vi "IETS_Tool_14_0805_bias_correct_neg_setpoints.vi"() -> ()   [LabVIEW 2013]
doc: "I. Description:\nThis example demonstrates how to continuously acquire and generate data at the same time, synchronized with one another.\n\nII. Instructions for Running:\n1. Select the physical channel to correspond to where your signal is input on the DAQ device. Also, select the corresponding channel for where your signal is being generated.\n2. Enter the minimum and maximum voltage ranges.\nNote: For better accuracy try to match the input range to the expected voltage level of the measured signal.\n3. Set the sample rate of the acquisition.\nNote: The rate should be at least twice as fast as the maximum frequency component of the signal being acquired. \n6. Select the Rate for the generation\n7. Select what type of signal to generate and the amplitude.\nNote: This example requires two DMA channels to run. If your hardware does not support two DMA channels, you need to set the Data Transfer Mechanism property for the Analog Output Task to use \"Interrupts\". The Data Transfer Mechanism property is located in the DAQmx Channel Property hierarchy at:\n\nDAQmx Channel Property Node>>Analog Output>>General Properties>>Advanced>>Data Transfer and Memory>>Data Transfer Mechanism\n\nRefer to your device documentation to determine how many DMA channels are supported for your hardware.\n\nIII. Block Diagram Steps:\n1. Create an analog input voltage channel. Also, create an analog output voltage channel.\n2. Set the rate for the sample clock. Additionally, define the sample mode to be continuous. Also, set the sample clock rate for the signal generation.\n2a. Call the Get Terminal Name with Device Prefix VI. This will take a Task and a terminal and create a properly formatted device + terminal name to use as the source of the Trigger.\n3. Define the parameters for a Digital Edge Start Trigger. Set the Analog output to trigger off the AI Start Trigger. This is an internal trigger signal.\n4. Use the Basic Function Generator VI to create the signal to be generated.\n5. Call the Start VI to arm the two functions. Make sure the analog output is armed before the analog input. This will ensure both will start at the same time.\n6. Read the waveform data in a loop until the user hits the stop button or an error occurs. The Is Task Done? VI is used to check for errors in the Analog Output Task.\n7. Call the Clear VI to Clear the Task\n8. Use the popup dialog box to display an error if any.\n\nIV. I/O Connections Overview:\nMake sure your signal input/output terminals match the Physical Channel I/O controls."
uses:
  <vilib>/Utility/error.llb/DialogType.ctl
  <vilib>/DAQmx/write.llb/DAQmx Write (Analog 2D DBL NChan NSamp).vi
  <vilib>/DAQmx/read.llb/DAQmx Read (Analog 1D DBL NChan 1Samp).vi
  <vilib>/DAQmx/write.llb/DAQmx Write (Analog DBL 1Chan 1Samp).vi
  <vilib>/DAQmx/read.llb/DAQmx Read (Analog DBL 1Chan 1Samp).vi
  <vilib>/Analysis/baseanly.llb/Mean (DBL).vi
  <vilib>/DAQmx/write.llb/DAQmx Write (Analog 1D DBL NChan 1Samp).vi
  <vilib>/DAQmx/create/channels.llb/DAQmx Create Channel (AO-Voltage-Basic).vi
  <vilib>/DAQmx/create/channels.llb/DAQmx Create Channel (AI-Voltage-Basic).vi
  <vilib>/DAQmx/configure/timing.llb/DAQmx Timing (Sample Clock).vi
  <vilib>/DAQmx/configure/trigger.llb/DAQmx Start Trigger (Digital Edge).vi
  <vilib>/DAQmx/miscellaneous.llb/DAQmx Fill In Error Info.vi
  <vilib>/Utility/file.llb/Write To Spreadsheet File (DBL).vi
  pid/pid.llb/PID (DBL).vi
  pid/pid.llb/PID Output Rate Limiter (DBL).vi
  <vilib>/ptbypt/NI_PtbyPt.lvlib
  <resource>/objmgr/daqmx.rc
  <vilib>/Analysis/NI_AALBase.lvlib
panel:
  in  "Bias Offset Correct":dbl
  out "Bias Sweep":dbl[](graph)
  out "element":dbl
  out "mean":dbl format="%.6f"
  out "size(s)":i32
  out "Numeric":i32
  in  "PID":bool=TRUE caption="Step Z"
  in  "Tab Control":enum32{"PID Controller", "Tapping Controls"}(tab)=enum."Tapping Controls"
  in  "Proportional Gain":dbl=0.0001
  in  "Integral Gain":dbl=1e-07
  in  "Differential Gain":dbl=1e-05
  in  "Setpoint":dbl=0.1
  in  "Piezo Delta rate":dbl=1000.0
  in  "Min Current":dbl=0.002
  in  "Max Current":dbl=10.2
  in  "Ramp Rate":dbl=20.0
  in  "Make Contact":i32=1200
  in  "Break Contact":i32=500
  in  "Step Length":i32=100
  in  "Step Max":dbl=0.3
  in  "Step Min":dbl=0.05
  out "Tapping Stop":bool
  out "Case":i32
  in  "Contact Cycles":i32
  in  "Tapping":bool caption="Step Z"
  out "x/y":dbl
  out "Waveform Chart":dbl(graph)
  in  "Piezo Control":dbl(slide) min=-10.0 max=10.0 step=0.001 scale=-10.0..10.0
  in  "Manual Z":bool caption="Step Z"
  in  "Sweep Amplitude":dbl=1.0
  in  "Stop Sweep":bool
  out "Connections 2":string="AI0=Current\nAI1=Bias\nAI2=dI/dV\nAI3=d2I/dV2\nAI4=X-Axis\nAI5=Z-Axis\n"
  out "Connections":string="AO0=Bias\nAO1=Z-axis\nAO2=X-Axis\nAO3=NA"
  out "Save Indicator":bool
  in  "Z-Direction":bool caption="Step Z"
  in  "Update Bias":bool
  in  "Save IV":bool
  in  "Save Decay":bool
  in  "Sweep Bias":bool
  in  "Step Z":bool
  in  "Comment":string="Molecule=TP4\nGain=10nA\nBias Gain=div/1\nSweep Freq.=0.0008Hz\nRef. Bias=4mV\nRef. Freq=2.977kHz\nGain LIA1=2mV\nTC LIA1=1s\nGain LIA2=5mV\nTC LIA2=1s\nLIA1=EGG\nLIA2=SRS\nEGG is driving(possible 5mV offset)"
  in  "Number Recorded":i32
  in  "DATA Filename":string="Data_"
  in  "Data Directory":path=path "E:/Research/Data"
  out "Current Decay":cluster{dbl[], dbl[]}(graph)
  out "d2I/dV2":cluster{dbl[], dbl[]}(graph)
  out "dI/dV":cluster{dbl[], dbl[]}(graph)
  out "IV":cluster{dbl[], dbl[]}(graph)
  in  "# Samples":i32=2000
  in  "Frequency (Hz)":dbl=1.0
  out "Measurement 2":cluster{i32, dbl, dbl[]}(graph) caption="Measurement"
  out "Actual Update Generation Rate 2":dbl=5000.0 caption="Actual Update Generation Rate" format="%0.2f"
  in  "stop 3":bool
  in  "Bias":dbl=0.1 caption="Bias Start Point" step=0.1 format="%_3g"
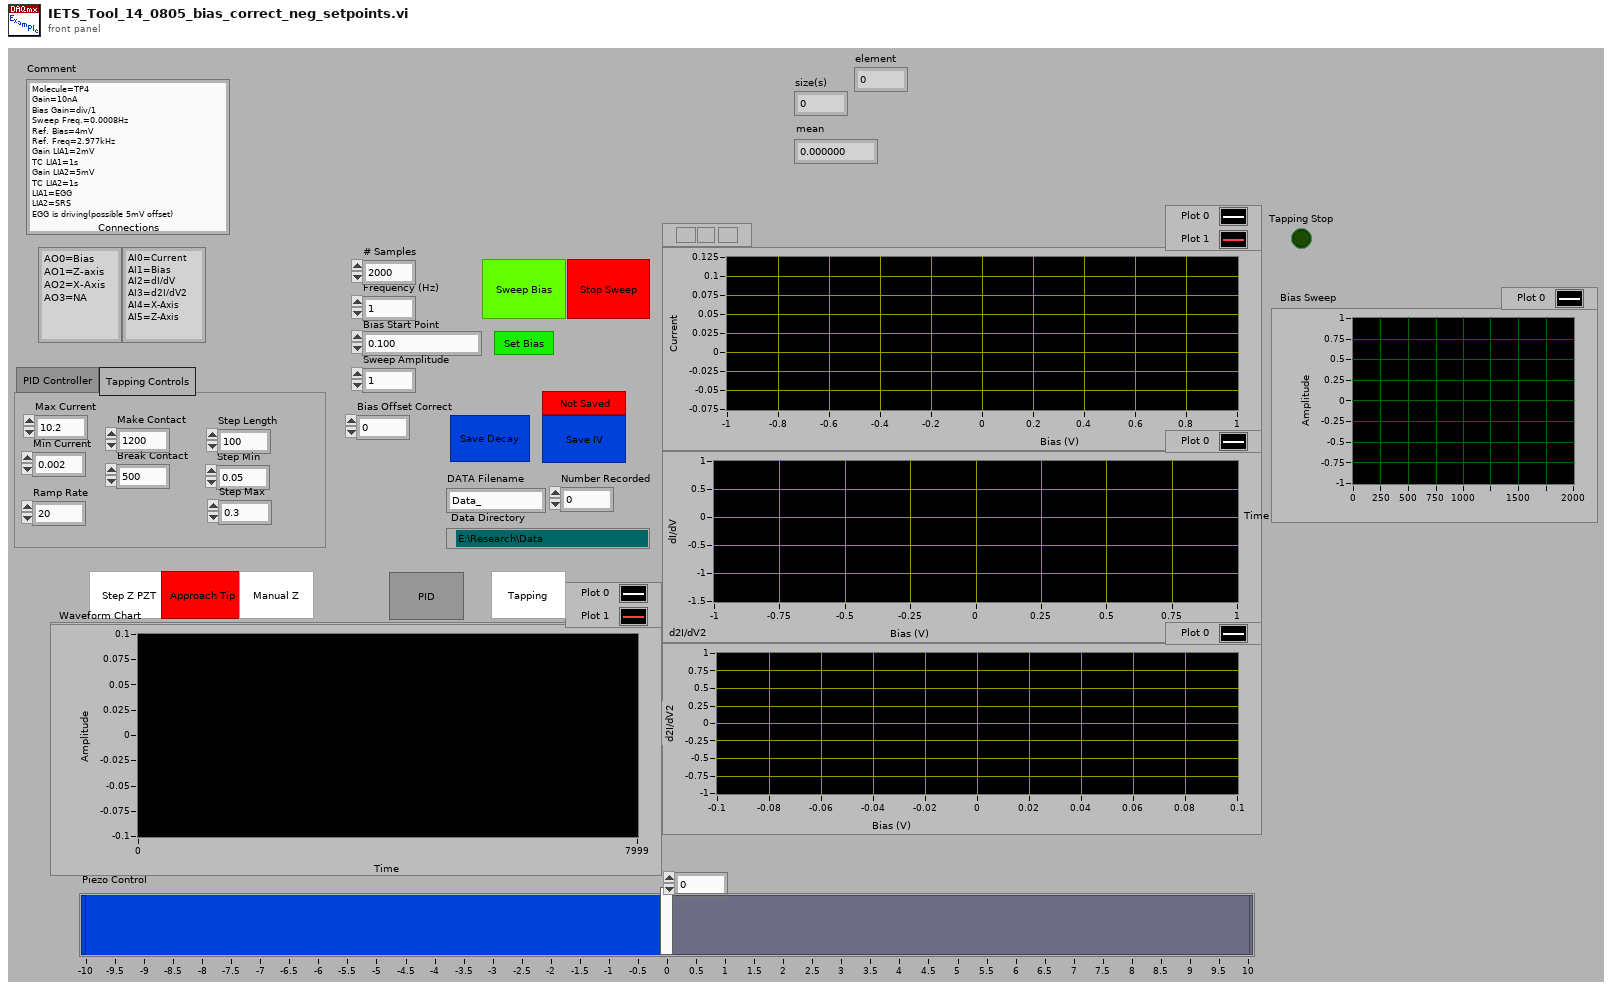
[diagram p1: front panel]
types:
  T1 = enum16{"open", "replace", "create", "open or create", "replace or create", "replace or create with confirmation"}
  T2 = typedef "DialogType.ctl" = u16
  T3 = cluster{"Proportional Gain":dbl, "Integral Gain ":dbl, "Differential Gain":dbl}
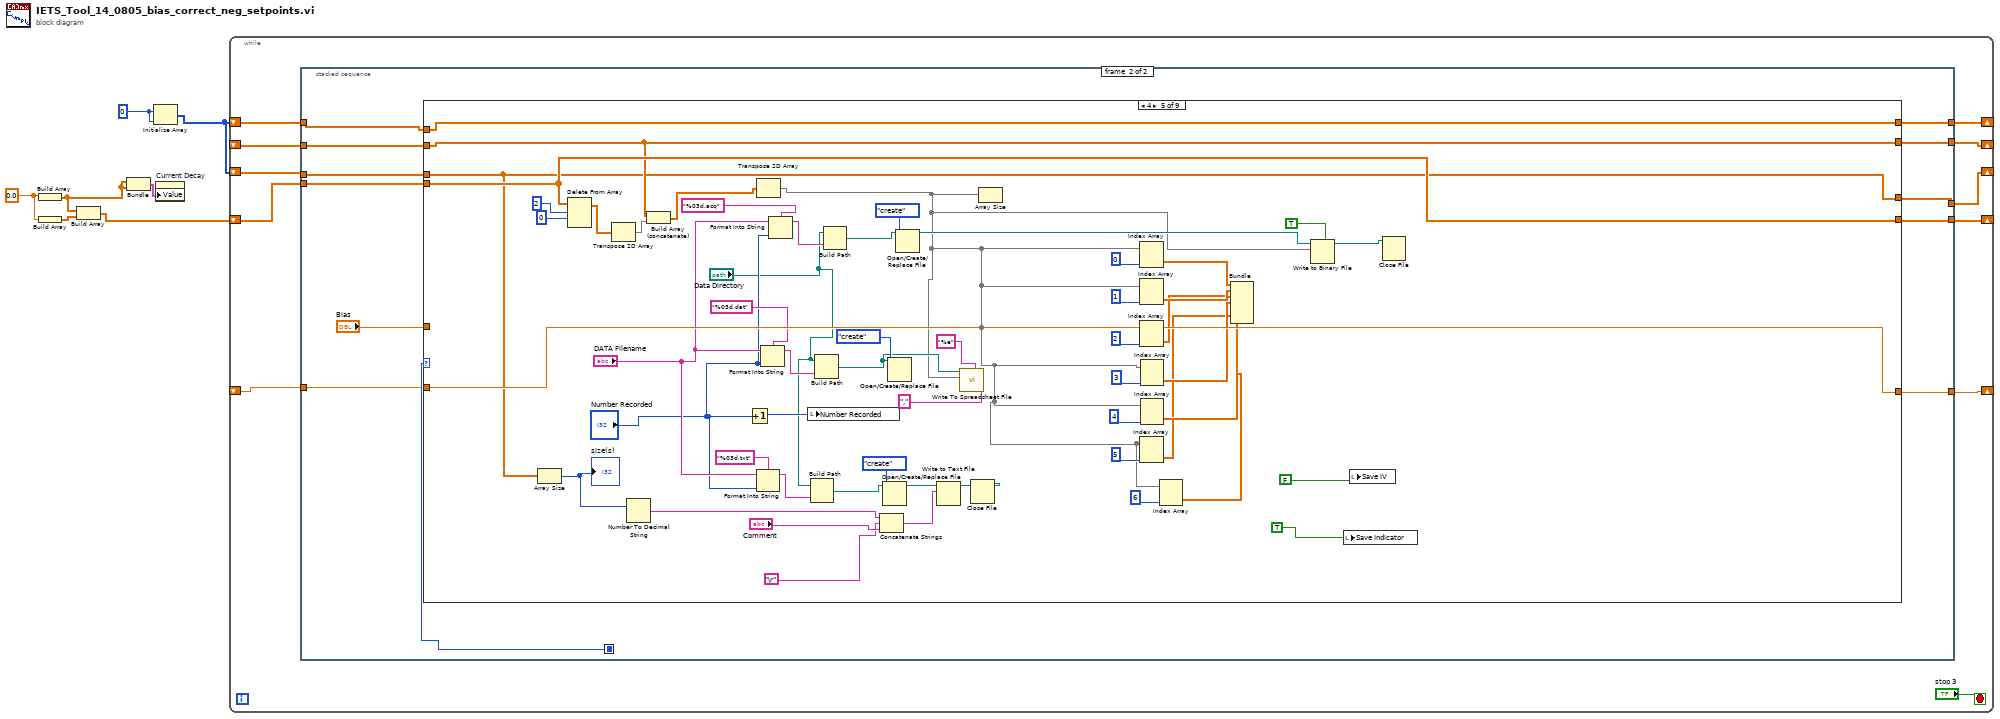
[diagram p0: block diagram]
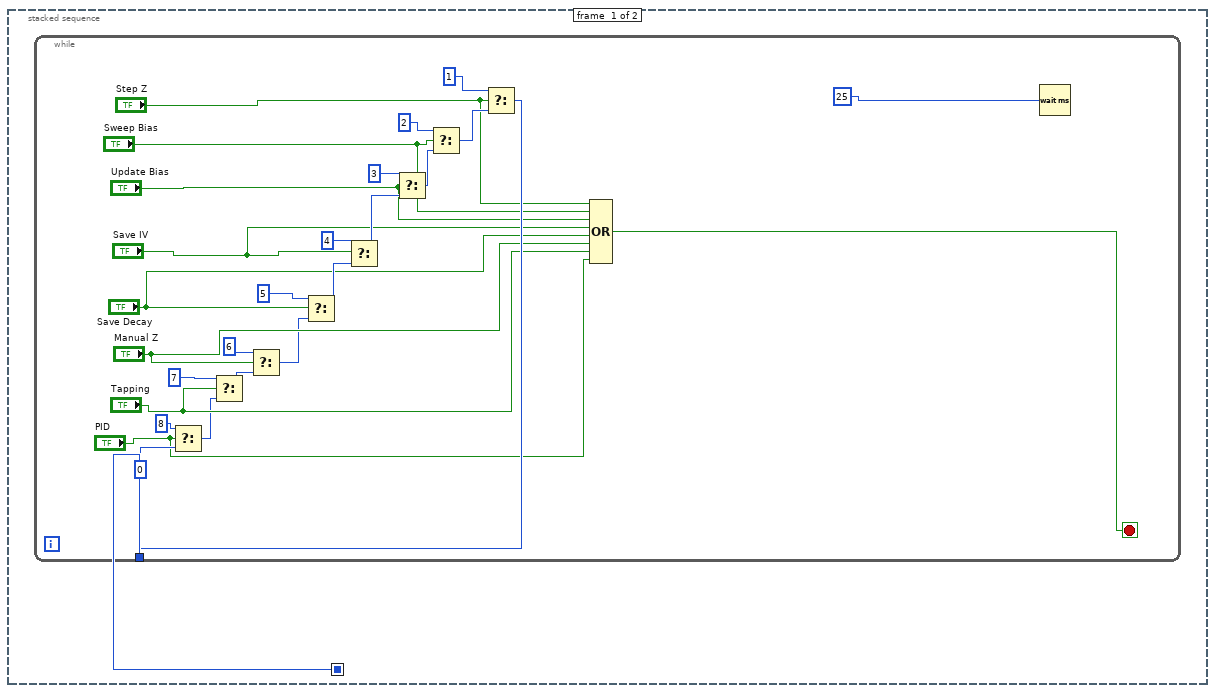
[diagram p2: hidden frame]
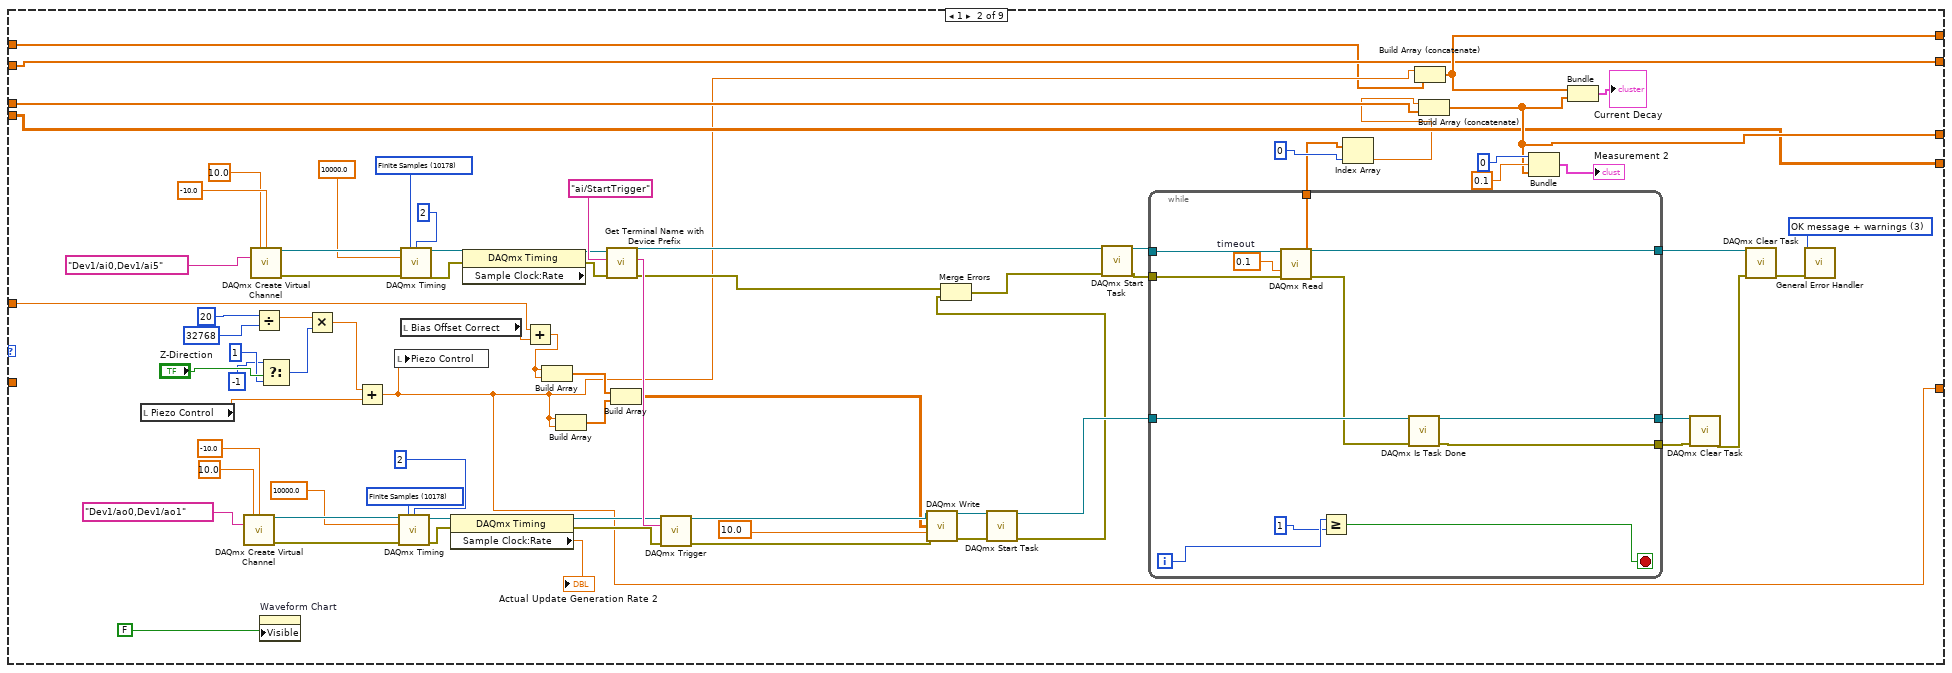
[diagram p4: hidden frame]
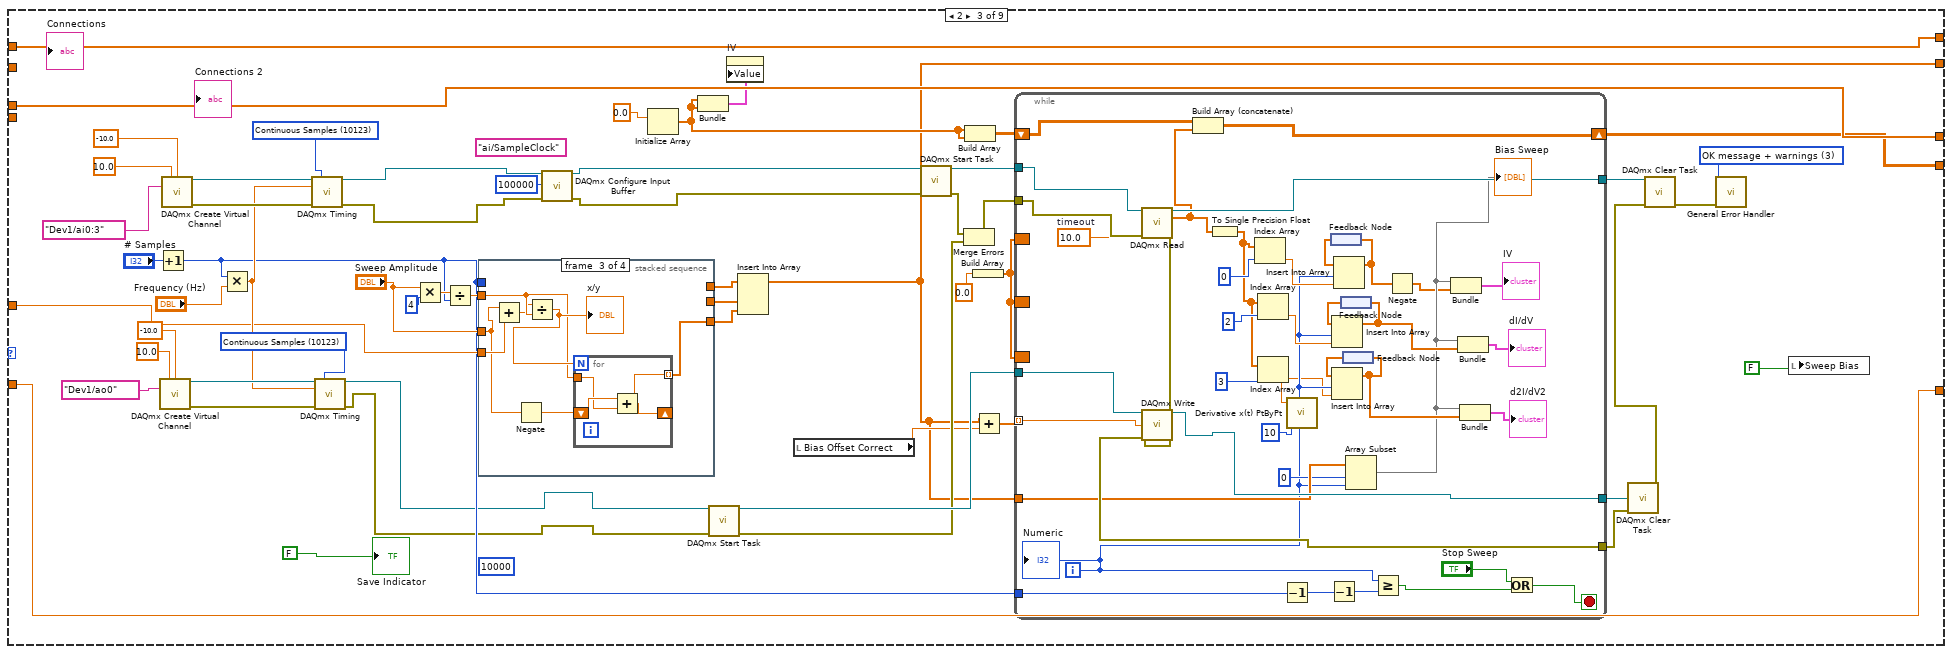
[diagram p5: hidden frame]
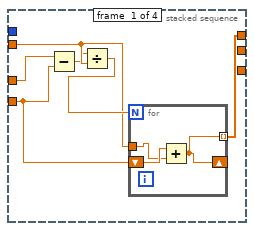
[diagram p6: hidden frame]
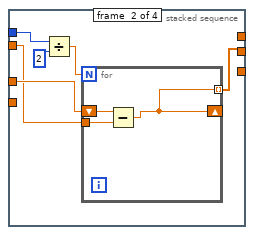
[diagram p7: hidden frame]
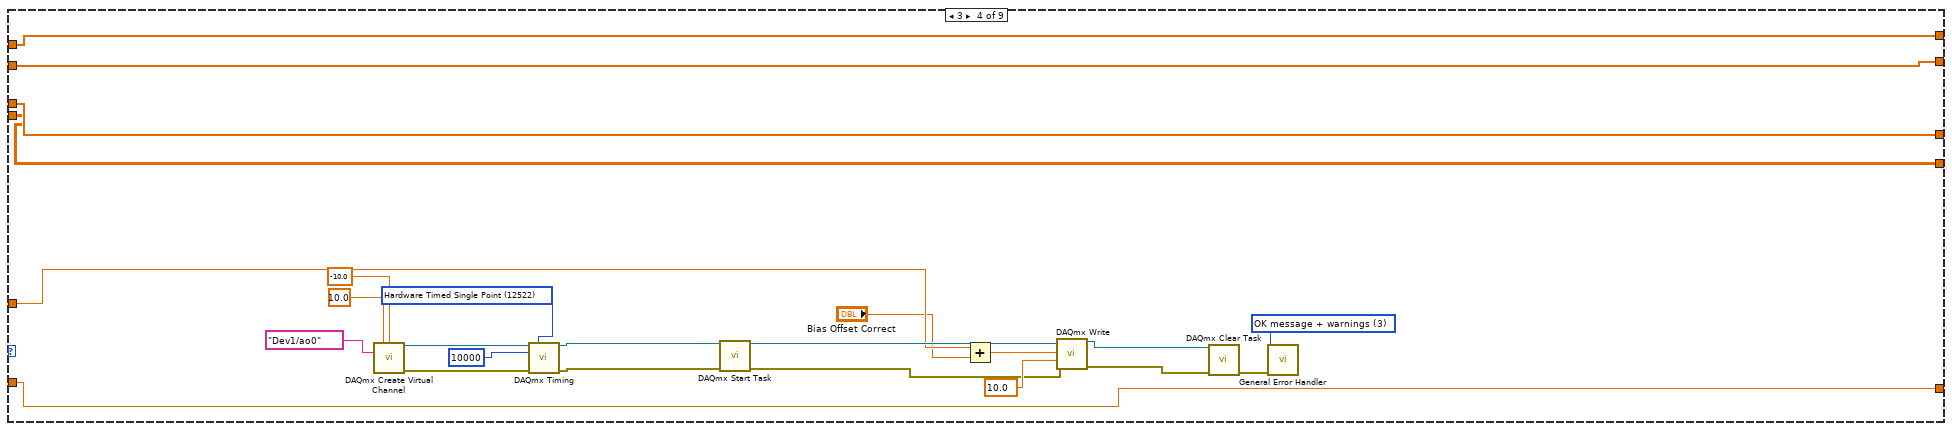
[diagram p9: hidden frame]
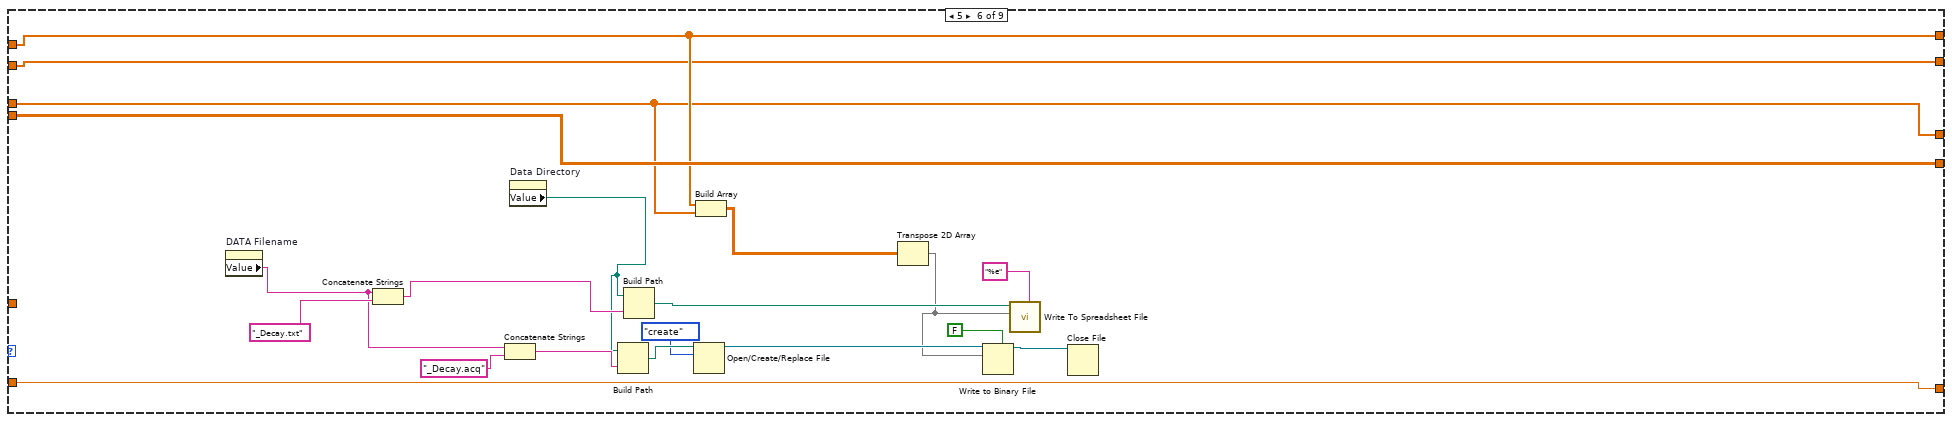
[diagram p10: hidden frame]
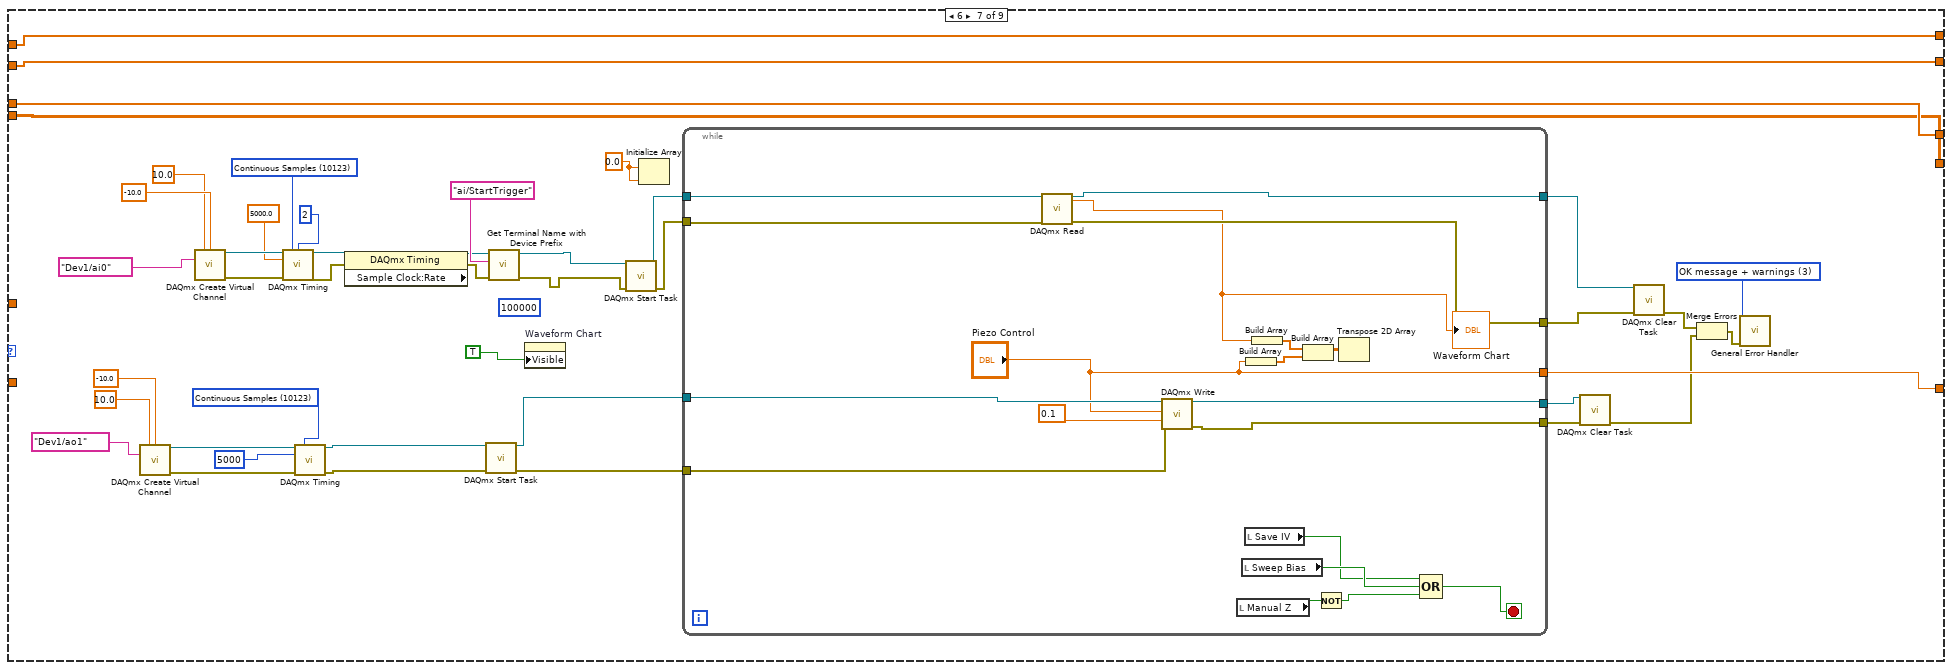
[diagram p11: hidden frame]
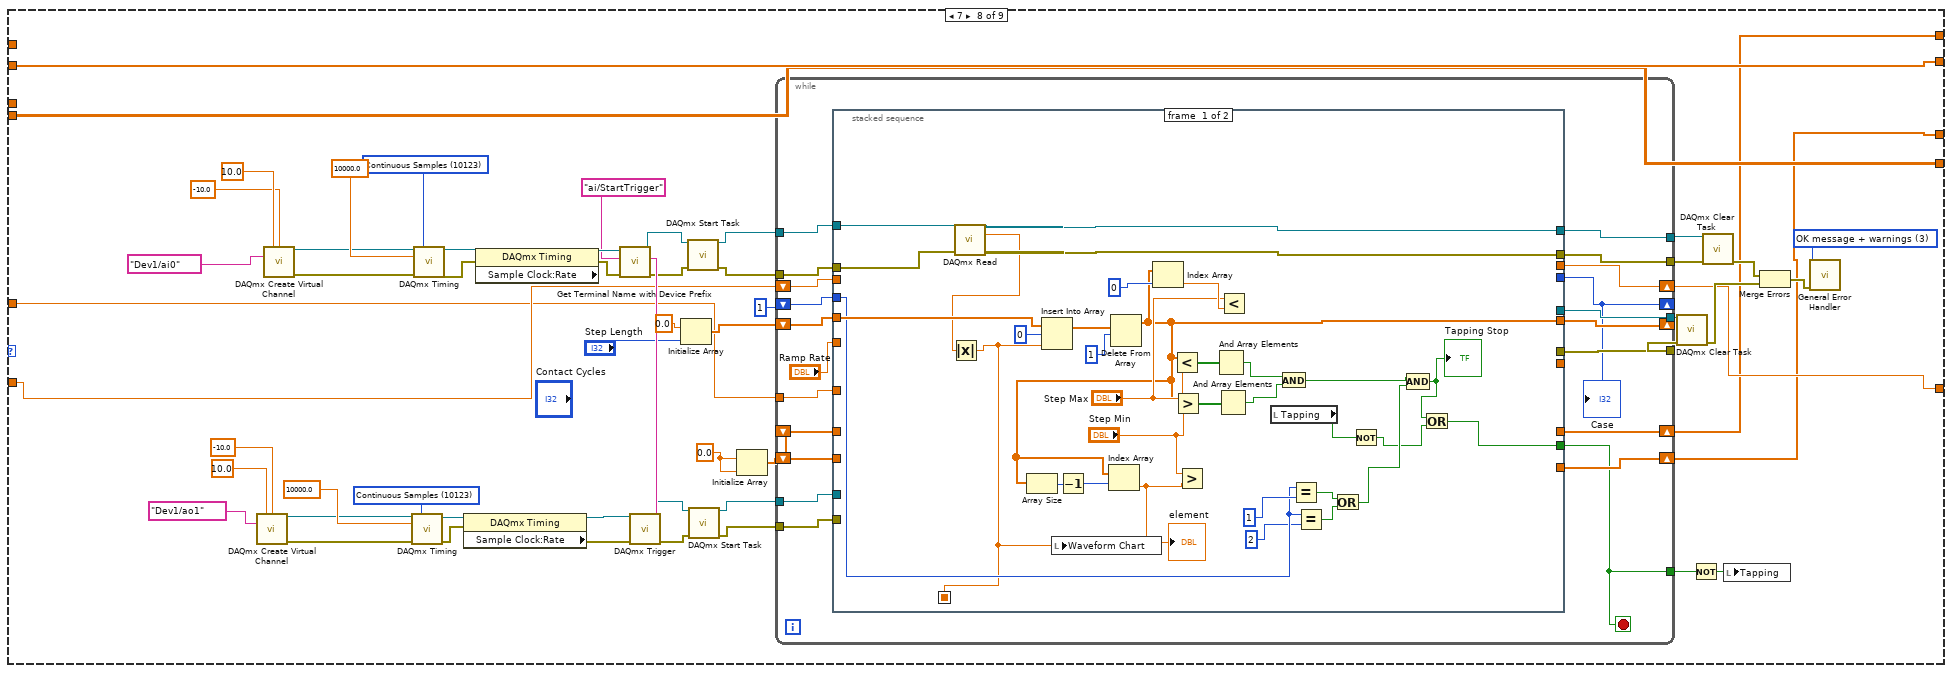
[diagram p12: hidden frame]
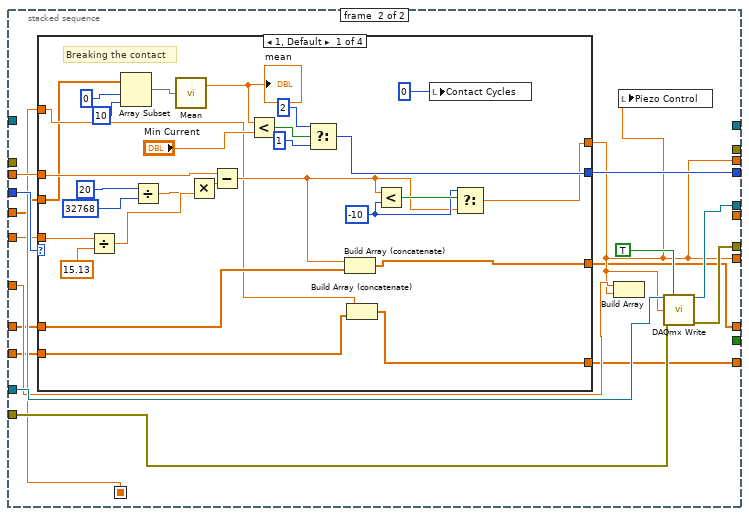
[diagram p13: hidden frame]
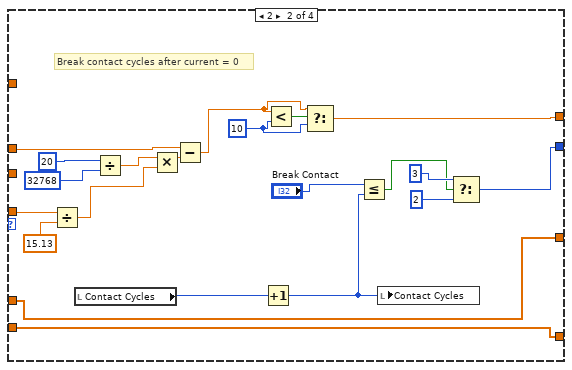
[diagram p14: hidden frame]
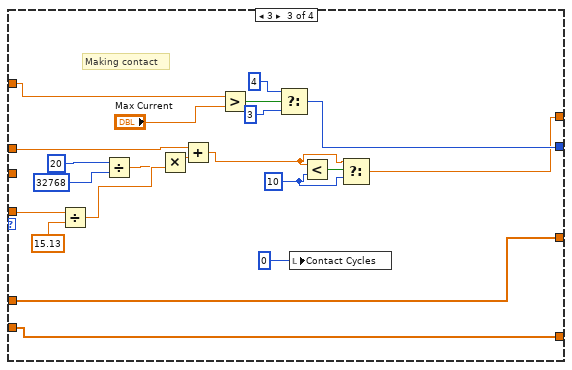
[diagram p15: hidden frame]
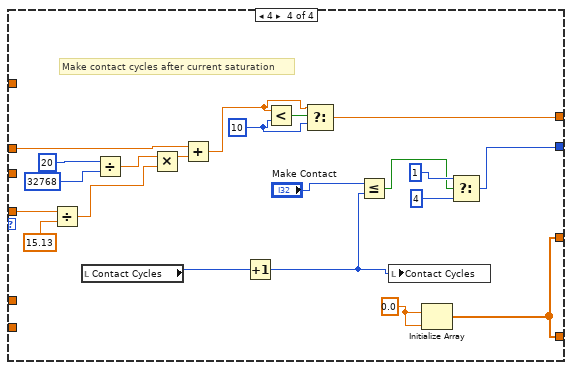
[diagram p16: hidden frame]
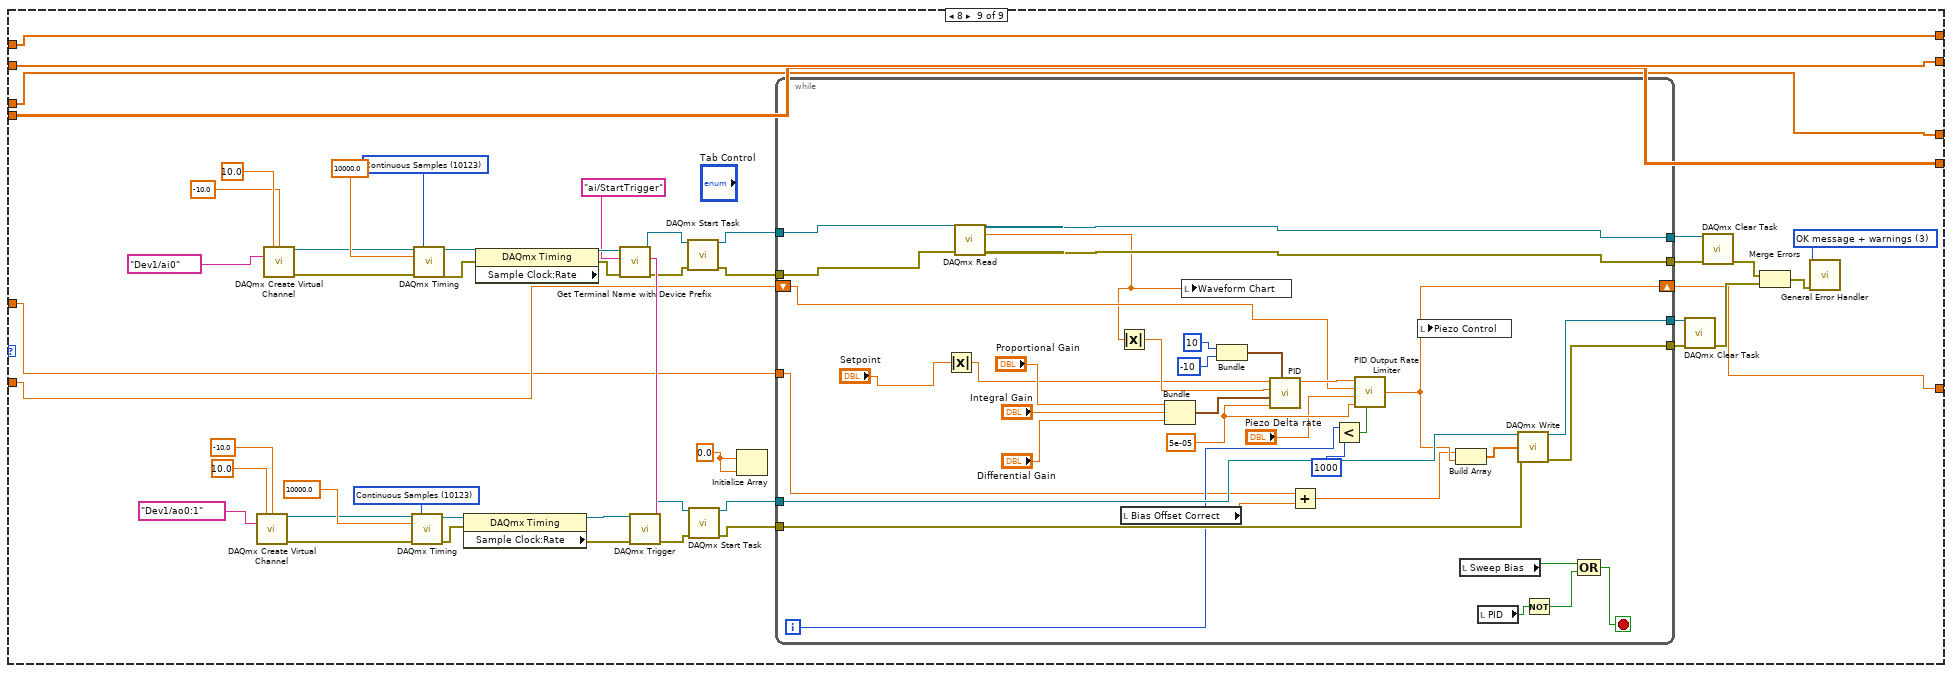
[diagram p17: hidden frame]
diagram:
  w2 = 0
  w7 = 0.0
  n1 = Build Array(w7) -> (w4:dbl[])
  n2 = Build Array(w7) -> (w6:dbl[])
  n3 = Build Array(w4, w6) -> (w5:dbl[][])
  n4 = Bundle(w4, w4) -> (w3:cluster{dbl[], dbl[]})  [unwired: 1 in]
  n5 = Initialize Array(w2, w2) -> (w1:i32[])
  n6 = property on="Current Decay" class="XYGraph (strict)"("Value"=w3) -> ()  [unwired: 2 in, 2 out]
  n7 = while {
    shift-right: [w16] -> _
    shift-left: w1 -> [w17]
    shift-right: [w14] -> _
    shift-left: w1 -> [w15]
    shift-right: [w12] -> _
    shift-left: _ -> [w13]
    shift-right: [w10] -> _
    shift-left: w5 -> [w11]
    shift-right: [w8] -> _
    shift-left: _ -> [w9]
    stop <- "stop 3" stop-if-true
    n8 = stacked-sequence {
      seq-local: [w19 _] -> [_ w58]
      tunnel: w17 -> [_ w57]
      tunnel: [_ w56] -> w16
      tunnel: w15 -> [_ w54]
      tunnel: [_ w53] -> w14
      tunnel: w13 -> [_ w52]
      tunnel: [_ w47] -> w12
      tunnel: w11 -> [_ w51]
      tunnel: [_ w50] -> w10
      tunnel: w9 -> [_ w49]
      tunnel: [_ w48] -> w8
      frame #0 {
        n9 = while {
          tunnel: [w37] -> w19
          stop <- w36 stop-if-true
          n10 = Select(t=8, s="PID", f=0) -> (s? t:f=w23:i32)
          n11 = Select(t=7, s="Tapping", f=w23) -> (s? t:f=w25:i32)
          n12 = Select(t=6, s="Manual Z", f=w25) -> (s? t:f=w26:i32)
          n13 = Select(t=5, s="Save Decay", f=w26) -> (s? t:f=w42:i32)
          n14 = Select(t=4, s="Save IV", f=w42) -> (s? t:f=w41:i32)
          n15 = Select(t=3, s="Update Bias", f=w41) -> (s? t:f=w39:i32)
          n16 = Select(t=2, s="Sweep Bias", f=w39) -> (s? t:f=w46:i32)
          n17 = Select(t=1, s="Step Z", f=w46) -> (s? t:f=w37:i32)
          n18 = Compound Arithmetic op=OR("Step Z", "Sweep Bias", "Update Bias", "Save IV", "Save Decay", "Manual Z", "Tapping", "PID") -> (w36:bool)
          n19 = Wait (ms)(milliseconds to wait=25) -> ()  [unwired: 1 out]
        }
      }
      frame #1 {
        n20 = case shown="4" w58 {
          tunnel: w57 -> [w63 w70 w191 w283 w303 w370 w415 _ w655]
          tunnel: [w63 w83 w191 w283 w303 w370 w415 w441 w655] -> w56
          tunnel: "Bias" -> [_ w66 w176 w277 _ _ _ w447 w654]
          tunnel: w54 -> [w62 w67 w188 w284 w350 w371 w417 _ w656]
          tunnel: [w62 w84 w188 w284 w350 w371 w417 w442 w656] -> w53
          tunnel: w52 -> [w61 _ w187 w282 w349 w372 _ w448 w663]
          tunnel: [w61 w68 w187 w282 w349 w372 w386 w443 w660] -> w47
          tunnel: w51 -> [w60 w81 _ w280 w329 w373 w414 w445 w661]
          tunnel: [w60 w81 w168 w280 w329 w373 w414 w445 w661] -> w50
          tunnel: [w59 w76 w151 w279 w327 w355 w416 w446 w662] -> w48
          tunnel: w49 -> [w59 w76 _ w279 w327 w355 w416 w446 w662]
          frame 0, Default {
          }
          frame 1 {
            w118 = T2 3 items=["no dialog", "OK message", "continue or stop message", "OK message + warnings", "continue/stop + warnings"] ("type of dialog (OK msg:1)")
            w130 = 10178 items=["Finite Samples"=10178, "Continuous Samples"=10123] ("sample mode")
            w135 = 10178 items=["Finite Samples"=10178, "Continuous Samples"=10123] ("sample mode")
            n21 = local read "Piezo Control"() -> (w71:dbl)
            n22 = call-poly <vilib>:"DAQmx Create Virtual Channel.vi"("maximum value"=10.0 ("maximum value 2"), "minimum value"=-10.0 ("minimum value 2"), "physical channels"=tag "Dev1/ao0,Dev1/ao1" ("physical channels 2")) -> ("task out"=w129:refnum<k21>, "error out"=w128:errorcluster)  [unwired: 11 in]
            n23 = call-poly <vilib>:"DAQmx Create Virtual Channel.vi"("maximum value"=10.0 ("Maximum Value 2"), "minimum value"=-10.0 ("Minimum Value 2"), "physical channels"=tag "Dev1/ai0,Dev1/ai5" ("Physical Channel 2")) -> ("task out"=w133:refnum<k21>, "error out"=w134:errorcluster)  [unwired: 11 in]
            n24 = Divide(x=20, y=32768) -> (x/y=w80:dbl)
            n25 = property on="Waveform Chart" class="WFChart (strict)"("Visible"=FALSE) -> ()  [unwired: 2 in, 2 out]
            n26 = Select(t=-1 ("f"), s="Z-Direction", f=1) -> (s? t:f=w78:i32)
            n27 = Multiply(x=w80, y=w78) -> (x*y=w79:dbl)
            n28 = Add(x=w79, y=w71) -> (x+y=w68:dbl)
            n29 = local write "Piezo Control"(w68) -> ()
            n30 = call-poly <vilib>:"DAQmx Timing.vi"("task/channels in"=w129, "sample mode"=w130, "samples per channel"=2, "rate"=10000.0 ("rate 2"), "error in"=w128) -> ("task out"=w113:refnum<k21>, "error out"=w112:errorcluster)  [unwired: 9 in]
            n31 = call-poly <vilib>:"DAQmx Timing.vi"("task/channels in"=w133, "sample mode"=w135, "samples per channel"=2, "rate"=10000.0 ("Rate 2"), "error in"=w134) -> ("task out"=w107:refnum<k21>, "error out"=w106:errorcluster)  [unwired: 9 in]
            n32 = local read "Bias Offset Correct"() -> (w65:dbl)
            n33 = property class="DAQmx Timing"(reference=w113, error in=w112) -> (reference out=w114:refnum<k21>, error out=w111:errorcluster, "Sample Clock:Rate"=→"Actual Update Generation Rate 2":dbl)
            n34 = property class="DAQmx Timing" props=["Sample Clock:Rate"](reference=w107, error in=w106) -> (reference out=w105:refnum<k21>, error out=w104:errorcluster)  [unwired: 1 out]
            n35 = Add(x=w66, y=w65) -> (x+y=w64:dbl)
            n36 = Build Array(w64, w64) -> (w91:dbl[])
            n37 = Build Array(w68, w68) -> (w90:dbl[])
            n38 = call "Get Terminal Name with Device Prefix.vi"("error in (no error)"=w104, "Local Terminal Name"="ai/StartTrigger" ("terminal"), "task/channels in"=w105) -> ("error out"=w110:errorcluster, "Terminal Name with Device Prefix"=w115:tag, "task out"=w95:refnum<k21>)  [unwired: 6 in]
            n39 = Build Array(w91, w90) -> (w89:dbl[][])
            n40 = call-poly <vilib>:"DAQmx Trigger.vi"("task/channels in"=w114, "source"=w115, "error in"=w111) -> ("task out"=w120:refnum<k21>, "error out"=w121:errorcluster)  [unwired: 11 in]
            n41 = call-poly <vilib>:"DAQmx Write.vi"("task/channels in"=w120, "data"=w89, "timeout"=10.0 ("Wirite Timeout"), "error in"=w121) -> ("task out"=w123:refnum<k21>, "error out"=w122:errorcluster)  [unwired: 9 in, 1 out]
            n42 = call <vilib>:"DAQmx Start Task.vi"("task/channels in"=w123, "error in"=w122) -> ("task out"=w127:refnum<k21>, "error out"=w109:errorcluster)  [unwired: 12 in]
            n43 = Merge Errors(w110, w109) -> (w97:errorcluster)
            n44 = call <vilib>:"DAQmx Start Task.vi"("task/channels in"=w95, "error in"=w97) -> ("task out"=w94:refnum<k21>, "error out"=w96:errorcluster)  [unwired: 12 in]
            n45 = while {
              tunnel: [w150] -> w136
              tunnel: w127 -> [w149]
              tunnel: [w148] -> w126
              tunnel: w94 -> [w139]
              tunnel: [w147] -> w103
              tunnel: [w144] -> w87
              tunnel: w96 -> [w140]
              i -> [w143]
              stop <- w141 stop-if-true
              w146 = 0.1  # timeout
              n46 = call-poly <vilib>:"DAQmx Read.vi"("task/channels in"=w139, "timeout"=w146, "error in"=w140) -> ("task out"=w150:refnum<k21>, "data"=w144:dbl[], "error out"=w145:errorcluster)  [unwired: 10 in]
              n47 = Greater Or Equal?(x=w143, y=1) -> (x >= y?=w141:bool)
              n48 = call <vilib>:"DAQmx Is Task Done.vi"("task/channels in"=w149, "error in"=w145) -> ("task out"=w148:refnum<k21>, "error out"=w147:errorcluster)  [unwired: 11 in, 1 out]
            }
            n49 = Index Array(array=w87, index=0) -> (element=w69:dbl)
            n50 = Build Array (concatenate)(w68, w67) -> (w84:dbl[])
            n51 = Build Array (concatenate)(w69, w70) -> (w83:dbl[])
            n52 = Bundle(0, 0.1, w83) -> (→"Measurement 2":cluster{i32, dbl, dbl[]})  [unwired: 1 in]
            n53 = Bundle(w84, w83) -> (→"Current Decay":cluster{dbl[], dbl[]})  [unwired: 1 in]
            n54 = call <vilib>:"DAQmx Clear Task.vi"("task in"=w126, "error in"=w103) -> ("error out"=w102:errorcluster)  [unwired: 13 in]
            n55 = call <vilib>:"DAQmx Clear Task.vi"("task in"=w136, "error in"=w102) -> ("error out"=w101:errorcluster)  [unwired: 13 in]
            n56 = call <vilib>:"General Error Handler.vi"("type of dialog (OK msg:1)"=w118, "error in (no error)"=w101) -> ()  [unwired: 9 in, 5 out]
          }
          frame 2 {
            (unwired) 10000
            w185 = 10123 items=["Finite Samples"=10178, "Continuous Samples"=10123, "Hardware Timed Single Point"=12522] ("sample mode")
            w186 = 10123 items=["Finite Samples"=10178, "Continuous Samples"=10123, "Hardware Timed Single Point"=12522] ("sample mode")
            (unwired) "ai/SampleClock" ("terminal")
            w196 = T2 3 items=["no dialog", "OK message", "continue or stop message", "OK message + warnings", "continue/stop + warnings"] ("type of dialog (OK msg:1)")
            n57 = Increment(x="# Samples") -> (x+1=w166:i32)
            n58 = call-poly <vilib>:"DAQmx Create Virtual Channel.vi"("maximum value"=10.0, "minimum value"=-10.0, "physical channels"=tag "Dev1/ao0") -> ("task out"=w199:refnum<k21>, "error out"=w198:errorcluster)  [unwired: 11 in]
            n59 = call-poly <vilib>:"DAQmx Create Virtual Channel.vi"("maximum value"=10.0 ("Maximum Value"), "minimum value"=-10.0 ("Minimum Value"), "physical channels"=tag "Dev1/ai0:3" ("Physical Channel")) -> ("task out"=w203:refnum<k21>, "error out"=w204:errorcluster)  [unwired: 11 in]
            n60 = Multiply(x=w166, y="Frequency (Hz)") -> (x*y=w190:dbl)
            n61 = call-poly <vilib>:"DAQmx Timing.vi"("task/channels in"=w203, "sample mode"=w185, "rate"=w190, "error in"=w204) -> ("task out"=w160:refnum<k21>, "error out"=w158:errorcluster)  [unwired: 10 in]
            n62 = call-poly <vilib>:"DAQmx Timing.vi"("task/channels in"=w199, "sample mode"=w186, "rate"=w190, "error in"=w198) -> ("task out"=w155:refnum<k21>, "error out"=w154:errorcluster)  [unwired: 10 in]
            n63 = Multiply(x="Sweep Amplitude", y=4) -> (x*y=w174:dbl)
            n64 = Divide(x=w174, y=w166) -> (x/y=w173:dbl)
            n65 = stacked-sequence {
              tunnel: "Sweep Amplitude" -> [w253 w259 w267 _]
              tunnel: w176 -> [w251 _ w271 _]
              tunnel: w173 -> [w249 w258 w269 _]
              tunnel: [w250 _ _ _] -> w172
              tunnel: w166 -> [_ w262 _ _]
              tunnel: [_ w257 _ _] -> w171
              tunnel: [_ _ w270 _] -> w170
              frame #0 {
                n66 = Subtract(x=w253, y=w251) -> (x-y=w248:dbl)
                n67 = Divide(x=w248, y=w249) -> (x/y=w252:dbl)
                n68 = for {
                  N: w252 -> [_]
                  tunnel: w249 -> [w255]
                  shift-right: [w254] -> _
                  shift-left: w251 -> [w256]
                  tunnel: [w254] -> w250 mode=indexing
                  n69 = Add(x=w256, y=w255) -> (x+y=w254:dbl)
                }
              }
              frame #1 {
                n70 = Divide(x=w262, y=2) -> (x/y=w260:dbl)
                n71 = for {
                  N: w260 -> [_]
                  tunnel: w258 -> [w264]
                  shift-right: [w263] -> _
                  shift-left: w259 -> [w265]
                  tunnel: [w263] -> w257 mode=indexing
                  n72 = Subtract(x=w265, y=w264) -> (x-y=w263:dbl)
                }
              }
              frame #2 {
                n73 = Add(x=w267, y=w271) -> (x+y=w268:dbl)
                n74 = Negate(x=w267) -> (-x=w266:dbl)
                n75 = Divide(x=w268, y=w269) -> (x/y=w272:dbl)
                "x/y" <- w272
                n76 = for {
                  N: w272 -> [_]
                  tunnel: w269 -> [w274]
                  shift-right: [w273] -> _
                  shift-left: w266 -> [w275]
                  tunnel: [w273] -> w270 mode=indexing
                  n77 = Add(x=w275, y=w274) -> (x+y=w273:dbl)
                }
              }
              frame #3 {
              }
            }
            n78 = call <vilib>:"DAQmx Configure Input Buffer.vi"("task/channels in"=w160, "buffer size (in samples per channel)"=100000, "error in"=w158) -> ("task out"=w159:refnum<k21>, "error out"=w157:errorcluster)  [unwired: 11 in]
            n79 = Initialize Array(0.0) -> (w165:dbl[])  [unwired: 1 in]
            n80 = Bundle(w165, w165) -> (w164:cluster{dbl[], dbl[]})  [unwired: 1 in]
            n81 = call <vilib>:"DAQmx Start Task.vi"("task/channels in"=w155, "error in"=w154) -> ("task out"=w184:refnum<k21>, "error out"=w180:errorcluster)  [unwired: 12 in]
            n82 = property on="IV" class="XYGraph (strict)"("Value"=w164) -> ()  [unwired: 2 in, 2 out]
            n83 = Insert Into Array(array=w172, new element #1=w171, new element #2=w170) -> (w151:dbl[])  [unwired: 1 in]
            n84 = local read "Bias Offset Correct"() -> (w152:dbl)
            n85 = call <vilib>:"DAQmx Start Task.vi"("task/channels in"=w159, "error in"=w157) -> ("task out"=w182:refnum<k21>, "error out"=w181:errorcluster)  [unwired: 12 in]
            n86 = Merge Errors(w181, w180) -> (w183:errorcluster)
            n87 = Build Array(w165, w165) -> (w167:dbl[][])
            n88 = Build Array(0.0) -> (w162:dbl[])
            n89 = Add(x=w151, y=w152) -> (x+y=w153:dbl[])
            n90 = while {
              tunnel: [w239] -> w205
              tunnel: [w242] -> w197
              tunnel: [w241] -> w194
              tunnel: w166 -> [w215]
              tunnel: w153 -> [w220] mode=indexing
              tunnel: w184 -> [w244]
              tunnel: w182 -> [w247]
              tunnel: w183 -> [w246]
              shift-right: [w221] -> w168
              shift-left: w167 -> [w240]
              tunnel: w151 -> [w237]
              border: w162 -> [_]
              border: w162 -> [_]
              border: w162 -> [_]
              i -> [w216]
              stop <- w217 stop-if-true
              w243 = 10.0  # timeout
              n91 = call-poly <vilib>:"DAQmx Read.vi"("task/channels in"=w247, "timeout"=w243, "error in"=w246) -> ("task out"=w239:refnum<k21>, "data"=w223:dbl[], "error out"=w245:errorcluster)  [unwired: 10 in]
              n92 = call-poly <vilib>:"DAQmx Write.vi"("task/channels in"=w244, "data"=w220, "error in"=w245) -> ("task out"=w242:refnum<k21>, "error out"=w241:errorcluster)  [unwired: 10 in, 1 out]
              n93 = Build Array (concatenate)(w240, w223) -> (w221:dbl[][])
              n94 = To Single Precision Float(number=w223) -> (single precision float=w222:sgl[])
              n95 = Index Array(array=w222, index=0) -> (element=w235:sgl)
              n96 = Index Array(array=w222, index=2) -> (element=w231:sgl)
              n97 = Index Array(array=w222, index=3) -> (element=w211:sgl)
              n98 = Decrement(x=w215) -> (x-1=w213:i32)
              n99 = call <vilib>:"Derivative x(t) PtByPt.vi"("dt"=10, "x"=w211) -> ()  [unwired: 2 in, 2 out]
              n100 = Decrement(x=w213) -> (x-1=w214:i32)
              n101 = feedback #1() -> (w234:dbl[])
              n102 = Insert Into Array(array=w234, index=w216, new element=w235) -> (w209:dbl[])
              n103 = feedback-in #1(w209) -> ()
              n104 = feedback #2() -> (w230:dbl[])
              n105 = Insert Into Array(array=w230, index=w216, new element=w231) -> (w228:dbl[])
              n106 = feedback-in #2(w228) -> ()
              n107 = feedback #3() -> (w229:dbl[])
              n108 = Insert Into Array(array=w229, index=w216, new element=w211) -> (w227:dbl[])
              n109 = feedback-in #3(w227) -> ()
              n110 = Array Subset(array=w237, index=0, length=w216) -> (w210:dbl[])
              "Bias Sweep" <- w210
              n111 = Greater Or Equal?(x=w216, y=w214) -> (x >= y?=w218:bool)
              n112 = Negate(x=w209) -> (-x=w208:dbl[])
              n113 = Bundle(w210, w208) -> (→"IV":cluster{dbl[], dbl[]})  [unwired: 1 in]
              n114 = Bundle(w210, w228) -> (→"dI/dV":cluster{dbl[], dbl[]})  [unwired: 1 in]
              n115 = Bundle(w210, w227) -> (→"d2I/dV2":cluster{dbl[], dbl[]})  [unwired: 1 in]
              n116 = Or(x="Stop Sweep", y=w218) -> (x .or. y?=w217:bool)
              "Numeric" <- w216
            }
            n117 = call <vilib>:"DAQmx Clear Task.vi"("task in"=w197, "error in"=w194) -> ("error out"=w193:errorcluster)  [unwired: 13 in]
            n118 = call <vilib>:"DAQmx Clear Task.vi"("task in"=w205, "error in"=w193) -> ("error out"=w192:errorcluster)  [unwired: 13 in]
            n119 = call <vilib>:"General Error Handler.vi"("type of dialog (OK msg:1)"=w196, "error in (no error)"=w192) -> ()  [unwired: 9 in, 5 out]
            n120 = local write "Sweep Bias"(FALSE) -> ()
            "Save Indicator" <- FALSE
          }
          frame 3 {
            w288 = T2 3 items=["no dialog", "OK message", "continue or stop message", "OK message + warnings", "continue/stop + warnings"] ("type of dialog (OK msg:1)")
            w293 = 12522 items=["Finite Samples"=10178, "Continuous Samples"=10123, "Hardware Timed Single Point"=12522] ("sample mode")
            n121 = call-poly <vilib>:"DAQmx Create Virtual Channel.vi"("maximum value"=10.0 ("maximum value 2"), "minimum value"=-10.0 ("minimum value 2"), "physical channels"=tag "Dev1/ao0" ("physical channels 2")) -> ("task out"=w296:refnum<k21>, "error out"=w295:errorcluster)  [unwired: 11 in]
            n122 = call-poly <vilib>:"DAQmx Timing.vi"("task/channels in"=w296, "sample mode"=w293, "rate"=10000, "error in"=w295) -> ("task out"=w292:refnum<k21>, "error out"=w291:errorcluster)  [unwired: 10 in]
            n123 = call <vilib>:"DAQmx Start Task.vi"("task/channels in"=w292, "error in"=w291) -> ("task out"=w290:refnum<k21>, "error out"=w289:errorcluster)  [unwired: 12 in]
            n124 = Add(x=w277, y="Bias Offset Correct") -> (x+y=w278:dbl)
            n125 = call-poly <vilib>:"DAQmx Write.vi"("task/channels in"=w290, "data"=w278, "timeout"=10.0 ("Wirite Timeout"), "error in"=w289) -> ("task out"=w286:refnum<k21>, "error out"=w285:errorcluster)  [unwired: 9 in, 1 out]
            n126 = call <vilib>:"DAQmx Clear Task.vi"("task in"=w286, "error in"=w285) -> ("error out"=w287:errorcluster)  [unwired: 13 in]
            n127 = call <vilib>:"General Error Handler.vi"("type of dialog (OK msg:1)"=w288, "error in (no error)"=w287) -> ()  [unwired: 9 in, 5 out]
          }
          frame 4 {
            n128 = Array Size(array=w303) -> (size(s)=w302:i32)
            "size(s)" <- w302
            n129 = Delete From Array(array=w329, length=2, index (row)=0) -> (array with subset deleted=w326:dbl[][])  [unwired: 1 in, 1 out]
            n130 = Transpose 2D Array(2D array=w326) -> (transposed array=w325:dbl[][])
            n131 = Number To Decimal String(number=w302) -> (decimal integer string=w301:string)  [unwired: 1 in]
            n132 = Build Array (concatenate)(w327, w325) -> (w307:dbl[][])
            n133 = Increment(x="Number Recorded") -> (x+1=w352:i32)
            n134 = Format Into String(format string="%03d.txt", initial string="DATA Filename", "Number Recorded") -> (resulting string=w340:string)  [unwired: 1 in, 1 out]
            n135 = Transpose 2D Array(2D array=w307) -> (transposed array=w306:dbl[][])
            n136 = Format Into String(format string="%03d.dat", initial string="DATA Filename", "Number Recorded") -> (resulting string=w354:string)  [unwired: 1 in, 1 out]
            n137 = Format Into String(format string="%03d.acq", initial string="DATA Filename", "Number Recorded") -> (resulting string=w347:string)  [unwired: 1 in, 1 out]
            n138 = local write "Number Recorded"(w352) -> ()
            n139 = Build Path(base path="Data Directory", name or relative path=w340) -> (appended path=w338:path)
            n140 = Build Path(base path="Data Directory", name or relative path=w354) -> (appended path=w351:path)
            n141 = Build Path(base path="Data Directory", name or relative path=w347) -> (appended path=w345:path)
            n142 = Concatenate Strings(w301, "\r", "Comment") -> (w323:string)
            n143 = Open/Create/Replace File(file path (use dialog)=w338, operation (0:open)=T1."create") -> (refnum out=w333:refnum<file>)  [unwired: 4 in, 2 out]
            n144 = Open/Create/Replace File(file path (use dialog)=w351, operation (0:open)=T1."create") -> ()  [unwired: 4 in, 3 out]
            n145 = Open/Create/Replace File(file path (use dialog)=w345, operation (0:open)=T1."create") -> (refnum out=w344:refnum<file>)  [unwired: 4 in, 2 out]
            n146 = Write to Text File(file (use dialog)=w333, text=w323) -> (refnum out=w332:refnum<file>)  [unwired: 2 in, 2 out]
            n147 = call-poly <vilib>:"Write To Spreadsheet File.vi"("delimiter (\\t)"=",", "format (%.3f)"="%e", "2D data"=w306, "file path (dialog if empty)"=w351) -> ()  [unwired: 4 in, 1 out]
            n148 = Close File(refnum=w332) -> ()  [unwired: 1 in, 2 out]
            n149 = Array Size(array=w306) -> ()  [unwired: 1 out]
            n150 = Index Array(array=w306, index (col)=0) -> (element=w315:dbl[])  [unwired: 1 in]
            n151 = Index Array(array=w306, index (col)=1) -> (element=w314:dbl[])  [unwired: 1 in]
            n152 = Index Array(array=w306, index (col)=2) -> (element=w313:dbl[])  [unwired: 1 in]
            n153 = Index Array(array=w306, index (col)=5) -> (element=w310:dbl[])  [unwired: 1 in]
            n154 = Index Array(array=w306, index (col)=3) -> (element=w312:dbl[])  [unwired: 1 in]
            n155 = Index Array(array=w306, index (col)=4) -> (element=w311:dbl[])  [unwired: 1 in]
            n156 = Index Array(array=w306, index (col)=6) -> (element=w309:dbl[])  [unwired: 1 in]
            n157 = Bundle(w315, w314, w313, w312, w311, w310, w309) -> ()  [unwired: 1 in, 1 out]
            n158 = Write to Binary File(file (use dialog)=w344, data=w306, 5:TRUE ("prepend array or string size? (T)")) -> (refnum out=w342:refnum<file>)  [unwired: 3 in, 2 out]
            n159 = local write "Save Indicator"(TRUE) -> ()
            n160 = local write "Save IV"(FALSE) -> ()
            n161 = Close File(refnum=w342) -> ()  [unwired: 1 in, 2 out]
          }
          frame 5 {
            n162 = property on="DATA Filename" class="Str"() -> ("Value"=w365:string)  [unwired: 2 in, 2 out]
            n163 = Concatenate Strings(w365, "_Decay.txt") -> (w369:string)
            n164 = Concatenate Strings(w365, "_Decay.acq") -> (w363:string)
            n165 = property on="Data Directory" class="Path"() -> ("Value"=w362:path)  [unwired: 2 in, 2 out]
            n166 = Build Path(base path=w362, name or relative path=w363) -> (appended path=w361:path)
            n167 = Build Path(base path=w362, name or relative path=w369) -> (appended path=w368:path)
            n168 = Open/Create/Replace File(file path (use dialog)=w361, operation (0:open)=T1."create") -> (refnum out=w367:refnum<file>)  [unwired: 4 in, 2 out]
            n169 = Build Array(w371, w370) -> (w358:dbl[][])
            n170 = Transpose 2D Array(2D array=w358) -> (transposed array=w357:dbl[][])
            n171 = Write to Binary File(file (use dialog)=w367, data=w357, 5:FALSE ("prepend array or string size? (T)")) -> (refnum out=w366:refnum<file>)  [unwired: 3 in, 2 out]
            n172 = call-poly <vilib>:"Write To Spreadsheet File.vi"("format (%.3f)"="%e", "2D data"=w357, "file path (dialog if empty)"=w368) -> ()  [unwired: 5 in, 1 out]
            n173 = Close File(refnum=w366) -> ()  [unwired: 1 in, 2 out]
          }
          frame 6 {
            (unwired) 100000
            w378 = 0.0
            w400 = 10123 items=["Finite Samples"=10178, "Continuous Samples"=10123] ("sample mode")
            w404 = T2 3 items=["no dialog", "OK message", "continue or stop message", "OK message + warnings", "continue/stop + warnings"] ("type of dialog (OK msg:1)")
            w408 = 10123 items=["Finite Samples"=10178, "Continuous Samples"=10123, "Hardware Timed Single Point"=12522] ("sample mode")
            n174 = call-poly <vilib>:"DAQmx Create Virtual Channel.vi"("maximum value"=10.0 ("maximum value 2"), "minimum value"=-10.0 ("minimum value 2"), "physical channels"=tag "Dev1/ao1" ("physical channels 2")) -> ("task out"=w410:refnum<k21>, "error out"=w409:errorcluster)  [unwired: 11 in]
            n175 = call-poly <vilib>:"DAQmx Create Virtual Channel.vi"("maximum value"=10.0 ("Maximum Value 2"), "minimum value"=-10.0 ("Minimum Value 2"), "physical channels"=tag "Dev1/ai0" ("Physical Channel 2")) -> ("task out"=w398:refnum<k21>, "error out"=w399:errorcluster)  [unwired: 11 in]
            n176 = call-poly <vilib>:"DAQmx Timing.vi"("task/channels in"=w398, "sample mode"=w400, "samples per channel"=2, "rate"=5000.0 ("Rate 2"), "error in"=w399) -> ("task out"=w394:refnum<k21>, "error out"=w393:errorcluster)  [unwired: 9 in]
            n177 = call-poly <vilib>:"DAQmx Timing.vi"("task/channels in"=w410, "sample mode"=w408, "rate"=5000, "error in"=w409) -> ("task out"=w407:refnum<k21>, "error out"=w406:errorcluster)  [unwired: 10 in]
            n178 = property class="DAQmx Timing" props=["Sample Clock:Rate"](reference=w394, error in=w393) -> (reference out=w392:refnum<k21>, error out=w391:errorcluster)  [unwired: 1 out]
            n179 = call <vilib>:"DAQmx Start Task.vi"("task/channels in"=w407, "error in"=w406) -> ("task out"=w405:refnum<k21>, "error out"=w387:errorcluster)  [unwired: 12 in]
            n180 = call "Get Terminal Name with Device Prefix.vi"("error in (no error)"=w391, "Local Terminal Name"="ai/StartTrigger" ("terminal"), "task/channels in"=w392) -> ("error out"=w375:errorcluster, "task out"=w376:refnum<k21>)  [unwired: 6 in, 1 out]
            n181 = property on="Waveform Chart" class="WFChart (strict)"("Visible"=TRUE) -> ()  [unwired: 2 in, 2 out]
            n182 = call <vilib>:"DAQmx Start Task.vi"("task/channels in"=w376, "error in"=w375) -> ("task out"=w385:refnum<k21>, "error out"=w389:errorcluster)  [unwired: 12 in]
            n183 = Initialize Array(w378, w378) -> ()  [unwired: 1 out]
            n184 = while {
              tunnel: w405 -> [w436]
              tunnel: w389 -> [w435]
              tunnel: w387 -> [w434]
              tunnel: ["Piezo Control"] -> w386
              tunnel: w385 -> [w433]
              tunnel: [w432] -> w384
              tunnel: [w431] -> w383
              tunnel: [w430] -> w381
              tunnel: [w424] -> w379
              stop <- w421 stop-if-true
              n185 = call-poly <vilib>:"DAQmx Read.vi"("task/channels in"=w433, "error in"=w435) -> ("task out"=w424:refnum<k21>, "data"=w419:dbl, "error out"=w430:errorcluster)  [unwired: 11 in]
              "Waveform Chart" <- w419
              n186 = call-poly <vilib>:"DAQmx Write.vi"("task/channels in"=w436, "data"="Piezo Control", "timeout"=0.1 ("Wirite Timeout"), "error in"=w434) -> ("task out"=w432:refnum<k21>, "error out"=w431:errorcluster)  [unwired: 9 in, 1 out]
              n187 = local read "Manual Z"() -> (w418:bool)
              n188 = local read "Sweep Bias"() -> (w422:bool)
              n189 = local read "Save IV"() -> (w420:bool)
              n190 = Build Array("Piezo Control") -> (w428:dbl[])
              n191 = Build Array(w419) -> (w427:dbl[])
              n192 = Build Array(w427, w428) -> (w426:dbl[][])
              n193 = Not(x=w418) -> (.not. x?=w423:bool)
              n194 = Transpose 2D Array(2D array=w426) -> ()  [unwired: 1 out]
              n195 = Compound Arithmetic op=OR(w420, w422, w423) -> (w421:bool)
            }
            n196 = call <vilib>:"DAQmx Clear Task.vi"("task in"=w384, "error in"=w383) -> ("error out"=w382:errorcluster)  [unwired: 13 in]
            n197 = call <vilib>:"DAQmx Clear Task.vi"("task in"=w379, "error in"=w381) -> ("error out"=w380:errorcluster)  [unwired: 13 in]
            n198 = Merge Errors(w380, w382) -> (w388:errorcluster)
            n199 = call <vilib>:"General Error Handler.vi"("type of dialog (OK msg:1)"=w404, "error in (no error)"=w388) -> ()  [unwired: 9 in, 5 out]
          }
          frame 7 {
            w440 = 0.0
            w461 = T2 3 items=["no dialog", "OK message", "continue or stop message", "OK message + warnings", "continue/stop + warnings"] ("type of dialog (OK msg:1)")
            w476 = 10123 items=["Finite Samples"=10178, "Continuous Samples"=10123] ("sample mode")
            w470 = 10123 items=["Finite Samples"=10178, "Continuous Samples"=10123] ("sample mode")
            n200 = call-poly <vilib>:"DAQmx Create Virtual Channel.vi"("maximum value"=10.0 ("maximum value 2"), "minimum value"=-10.0 ("minimum value 2"), "physical channels"=tag "Dev1/ao1" ("physical channels 2")) -> ("task out"=w477:refnum<k21>, "error out"=w478:errorcluster)  [unwired: 11 in]
            n201 = call-poly <vilib>:"DAQmx Create Virtual Channel.vi"("maximum value"=10.0 ("Maximum Value 2"), "minimum value"=-10.0 ("Minimum Value 2"), "physical channels"=tag "Dev1/ai0" ("Physical Channel 2")) -> ("task out"=w472:refnum<k21>, "error out"=w471:errorcluster)  [unwired: 11 in]
            n202 = call-poly <vilib>:"DAQmx Timing.vi"("task/channels in"=w477, "sample mode"=w476, "rate"=10000.0 ("rate 2"), "error in"=w478) -> ("task out"=w485:refnum<k21>, "error out"=w486:errorcluster)  [unwired: 10 in]
            n203 = call-poly <vilib>:"DAQmx Timing.vi"("task/channels in"=w472, "sample mode"=w470, "rate"=10000.0 ("Rate 2"), "error in"=w471) -> ("task out"=w488:refnum<k21>, "error out"=w489:errorcluster)  [unwired: 10 in]
            n204 = property class="DAQmx Timing" props=["Sample Clock:Rate"](reference=w485, error in=w486) -> (reference out=w484:refnum<k21>, error out=w487:errorcluster)  [unwired: 1 out]
            n205 = property class="DAQmx Timing" props=["Sample Clock:Rate"](reference=w488, error in=w489) -> (reference out=w490:refnum<k21>, error out=w491:errorcluster)  [unwired: 1 out]
            n206 = call "Get Terminal Name with Device Prefix.vi"("error in (no error)"=w491, "Local Terminal Name"="ai/StartTrigger" ("terminal"), "task/channels in"=w490) -> ("error out"=w459:errorcluster, "Terminal Name with Device Prefix"=w483:tag, "task out"=w457:refnum<k21>)  [unwired: 6 in]
            n207 = call-poly <vilib>:"DAQmx Trigger.vi"("task/channels in"=w484, "source"=w483, "error in"=w487) -> ("task out"=w452:refnum<k21>, "error out"=w449:errorcluster)  [unwired: 11 in]
            n208 = Initialize Array(0.0, "Step Length") -> (w455:dbl[])
            n209 = call <vilib>:"DAQmx Start Task.vi"("task/channels in"=w457, "error in"=w459) -> ("task out"=w456:refnum<k21>, "error out"=w458:errorcluster)  [unwired: 12 in]
            n210 = call <vilib>:"DAQmx Start Task.vi"("task/channels in"=w452, "error in"=w449) -> ("task out"=w451:refnum<k21>, "error out"=w450:errorcluster)  [unwired: 12 in]
            n211 = Initialize Array(w440, w440) -> (w439:dbl[])
            n212 = while {
              tunnel: w456 -> [w512]
              tunnel: w458 -> [w511]
              tunnel: w451 -> [w510]
              tunnel: w450 -> [w509]
              tunnel: [w508] -> w467
              tunnel: [w507] -> w466
              tunnel: [w506] -> w464
              tunnel: [w505] -> w462
              shift-right: [w503] -> _
              shift-left: w455 -> [w504]
              tunnel: w447 -> [w501]
              shift-right: [w500] -> _
              shift-left: 1 -> [w499]
              shift-right: [w498] -> w443
              shift-left: w448 -> [w502]
              shift-right: [w496] -> w442
              shift-left: w439 -> [w497]
              shift-right: [w494] -> w441
              shift-left: w439 -> [w495]
              tunnel: [w492] -> w438
              stop <- w492 stop-if-true
              n213 = stacked-sequence {
                seq-local: [w514 _] -> [_ w554]
                tunnel: w512 -> [w545 _]
                tunnel: w511 -> [w544 _]
                tunnel: w510 -> [_ w562]
                tunnel: w509 -> [_ w561]
                tunnel: [w542 _] -> w508
                tunnel: [w543 _] -> w507
                tunnel: [_ w559] -> w506
                tunnel: [_ w560] -> w505
                tunnel: w504 -> [w539 w546]
                tunnel: [w522 _] -> w503
                tunnel: [w515 _] -> w492
                tunnel: w502 -> [_ w558]
                tunnel: w501 -> [_ w557]
                tunnel: [_ w556] -> w500
                tunnel: w499 -> [w531 w555]
                tunnel: "Ramp Rate" -> [_ w553]
                tunnel: [_ w551] -> _
                tunnel: [_ w551] -> w498
                tunnel: w497 -> [_ w550]
                tunnel: [_ w549] -> w496
                tunnel: w495 -> [_ w548]
                tunnel: [_ w547] -> w494
                frame #0 {
                  n214 = call-poly <vilib>:"DAQmx Read.vi"("task/channels in"=w545, "error in"=w544) -> ("task out"=w542:refnum<k21>, "data"=w513:dbl, "error out"=w543:errorcluster)  [unwired: 11 in]
                  n215 = Absolute Value(x=w513) -> (abs(x)=w514:dbl)
                  n216 = Insert Into Array(array=w539, index=0, new element=w514) -> (w540:dbl[])
                  n217 = local write "Waveform Chart"(w514) -> ()
                  n218 = Delete From Array(array=w540, length=1) -> (array with subset deleted=w522:dbl[])  [unwired: 1 in, 1 out]
                  n219 = Array Size(array=w522) -> (size(s)=w532:i32)
                  n220 = Decrement(x=w532) -> (x-1=w523:i32)
                  n221 = Index Array(array=w522, index=w523) -> (element=w525:dbl)
                  "element" <- w525
                  n222 = Index Array(array=w522, index=0) -> (element=w527:dbl)
                  n223 = Less?(x=w522, y="Step Max") -> (x < y?=w537:bool[])
                  n224 = Greater?(x=w522, y="Step Min") -> (0:w536:bool[])
                  n225 = Greater?(x="Step Min", y=w525) -> ()  [unwired: 1 out]
                  n226 = And Array Elements(Boolean array=w537) -> (logical AND=w521:bool)
                  n227 = And Array Elements(Boolean array=w536) -> (logical AND=w520:bool)
                  n228 = Less?(x="Step Max", y=w527) -> ()  [unwired: 1 out]
                  n229 = local read "Tapping"() -> (w517:bool)
                  n230 = And(x=w521, y=w520) -> (x .and. y?=w535:bool)
                  n231 = Equal?(x=w531, y=1) -> (x = y?=w529:bool)
                  n232 = Equal?(x=w531, y=2) -> (x = y?=w528:bool)
                  n233 = Or(x=w529, y=w528) -> (x .or. y?=w519:bool)
                  n234 = Not(x=w517) -> (.not. x?=w516:bool)
                  n235 = Compound Arithmetic op=AND(w535, w519) -> (w518:bool)
                  "Tapping Stop" <- w518
                  n236 = Or(x=w518, y=w516) -> (x .or. y?=w515:bool)
                }
                frame #1 {
                  n237 = case shown="1, Default" w555 {
                    tunnel: [w570 w593 w614 w640] -> w551
                    tunnel: w558 -> [w583 w595 w625 w637]
                    tunnel: [w578 w594 w619 w636] -> w556
                    tunnel: w554 -> [w569 _ w624 _]
                    tunnel: w553 -> [w584 w598 w626 w635]
                    tunnel: w550 -> [w574 w592 w613 _]
                    tunnel: [w576 w592 w613 w633] -> w549
                    tunnel: w548 -> [w568 w591 w612 _]
                    tunnel: [w575 w591 w612 w633] -> w547
                    tunnel: w546 -> [w567 _ _ _]
                    frame 1, Default {
                      w572 = -10
                      # "Breaking the contact"
                      n238 = Divide(x=w584, y=15.13) -> (x/y=w588:dbl)
                      n239 = Array Subset(array=w567, index=0, length=10) -> (w564:dbl[])
                      n240 = Divide(x=20, y=32768) -> (x/y=w585:dbl)
                      n241 = call-poly <vilib>:"Mean.vi"("X"=w564) -> ("mean"=w563:dbl)  [unwired: 1 out]
                      "mean" <- w563
                      n242 = Multiply(x=w585, y=w588) -> (x*y=w590:dbl)
                      n243 = Subtract(x=w583, y=w590) -> (x-y=w571:dbl)
                      n244 = Less?(x=w563, y="Min Current") -> (x < y?=w581:bool)
                      n245 = Select(t=2, s=w581, f=1) -> (s? t:f=w578:i32)
                      n246 = Build Array (concatenate)(w571, w574) -> (w576:dbl[])
                      n247 = Build Array (concatenate)(w569, w568) -> (w575:dbl[])
                      n248 = Less?(x=w571, y=w572) -> (x < y?=w573:bool)
                      n249 = local write "Contact Cycles"(0) -> ()
                      n250 = Select(t=w572, s=w573, f=w571) -> (s? t:f=w570:dbl)
                    }
                    frame 2 {
                      w610 = 10
                      # "Break contact cycles after current = 0"
                      n251 = Divide(x=w598, y=15.13) -> (x/y=w606:dbl)
                      n252 = local read "Contact Cycles"() -> (w597:i32)
                      n253 = Divide(x=20, y=32768) -> (x/y=w599:dbl)
                      n254 = Multiply(x=w599, y=w606) -> (x*y=w608:dbl)
                      n255 = Subtract(x=w595, y=w608) -> (x-y=w600:dbl)
                      n256 = Increment(x=w597) -> (x+1=w596:i32)
                      n257 = Less?(x=w600, y=w610) -> (x < y?=w609:bool)
                      n258 = Select(t=w600, s=w609, f=w610) -> (s? t:f=w593:dbl)
                      n259 = Less Or Equal?(x="Break Contact", y=w596) -> (x <= y?=w603:bool)
                      n260 = local write "Contact Cycles"(w596) -> ()
                      n261 = Select(t=3, s=w603, f=2) -> (s? t:f=w594:i32)
                    }
                    frame 3 {
                      w617 = 10
                      # "Making contact"
                      n262 = Divide(x=w626, y=15.13) -> (x/y=w630:dbl)
                      n263 = Divide(x=20, y=32768) -> (x/y=w627:dbl)
                      n264 = Multiply(x=w627, y=w630) -> (x*y=w632:dbl)
                      n265 = Add(x=w625, y=w632) -> (x+y=w615:dbl)
                      n266 = Greater?(x=w624, y="Max Current") -> (0:w622:bool)
                      n267 = Select(t=4, s=w622, f=3) -> (s? t:f=w619:i32)
                      n268 = local write "Contact Cycles"(0) -> ()
                      n269 = Less?(x=w615, y=w617) -> (x < y?=w616:bool)
                      n270 = Select(t=w615, s=w616, f=w617) -> (s? t:f=w614:dbl)
                    }
                    frame 4 {
                      w634 = 0.0
                      w652 = 10
                      # "Make contact cycles after current saturation"
                      n271 = Divide(x=w635, y=15.13) -> (x/y=w648:dbl)
                      n272 = local read "Contact Cycles"() -> (w642:i32)
                      n273 = Divide(x=20, y=32768) -> (x/y=w638:dbl)
                      n274 = Multiply(x=w638, y=w648) -> (x*y=w650:dbl)
                      n275 = Add(x=w637, y=w650) -> (x+y=w639:dbl)
                      n276 = Increment(x=w642) -> (x+1=w641:i32)
                      n277 = Less?(x=w639, y=w652) -> (x < y?=w651:bool)
                      n278 = Select(t=w639, s=w651, f=w652) -> (s? t:f=w640:dbl)
                      n279 = Less Or Equal?(x="Make Contact", y=w641) -> (x <= y?=w645:bool)
                      n280 = local write "Contact Cycles"(w641) -> ()
                      n281 = Initialize Array(w634, w634) -> (w633:dbl[])
                      n282 = Select(t=1, s=w645, f=4) -> (s? t:f=w636:i32)
                    }
                  }
                  n283 = Build Array(w557, w551) -> ()  [unwired: 1 out]
                  n284 = local write "Piezo Control"(w551) -> ()
                  n285 = call-poly <vilib>:"DAQmx Write.vi"("task/channels in"=w562, "auto start"=TRUE, "data"=w551, "error in"=w561) -> ("task out"=w560:refnum<k21>, "error out"=w559:errorcluster)  [unwired: 9 in, 1 out]
                }
              }
              "Case" <- w500
            }
            n286 = call <vilib>:"DAQmx Clear Task.vi"("task in"=w462, "error in"=w464) -> ("error out"=w463:errorcluster)  [unwired: 13 in]
            n287 = Not(x=w438) -> (.not. x?=w437:bool)
            n288 = call <vilib>:"DAQmx Clear Task.vi"("task in"=w467, "error in"=w466) -> ("error out"=w465:errorcluster)  [unwired: 13 in]
            n289 = local write "Tapping"(w437) -> ()
            n290 = Merge Errors(w465, w463) -> (w460:errorcluster)
            n291 = call <vilib>:"General Error Handler.vi"("type of dialog (OK msg:1)"=w461, "error in (no error)"=w460) -> ()  [unwired: 9 in, 5 out]
          }
          frame 8 {
            w659 = 0.0
            w673 = T2 3 items=["no dialog", "OK message", "continue or stop message", "OK message + warnings", "continue/stop + warnings"] ("type of dialog (OK msg:1)")
            w686 = 10123 items=["Finite Samples"=10178, "Continuous Samples"=10123] ("sample mode")
            w680 = 10123 items=["Finite Samples"=10178, "Continuous Samples"=10123] ("sample mode")
            n292 = call-poly <vilib>:"DAQmx Create Virtual Channel.vi"("maximum value"=10.0 ("maximum value 2"), "minimum value"=-10.0 ("minimum value 2"), "physical channels"=tag "Dev1/ao0:1" ("physical channels 2")) -> ("task out"=w687:refnum<k21>, "error out"=w688:errorcluster)  [unwired: 11 in]
            n293 = call-poly <vilib>:"DAQmx Create Virtual Channel.vi"("maximum value"=10.0 ("Maximum Value 2"), "minimum value"=-10.0 ("Minimum Value 2"), "physical channels"=tag "Dev1/ai0" ("Physical Channel 2")) -> ("task out"=w682:refnum<k21>, "error out"=w681:errorcluster)  [unwired: 11 in]
            n294 = call-poly <vilib>:"DAQmx Timing.vi"("task/channels in"=w687, "sample mode"=w686, "rate"=10000.0 ("rate 2"), "error in"=w688) -> ("task out"=w695:refnum<k21>, "error out"=w696:errorcluster)  [unwired: 10 in]
            n295 = call-poly <vilib>:"DAQmx Timing.vi"("task/channels in"=w682, "sample mode"=w680, "rate"=10000.0 ("Rate 2"), "error in"=w681) -> ("task out"=w698:refnum<k21>, "error out"=w699:errorcluster)  [unwired: 10 in]
            n296 = property class="DAQmx Timing" props=["Sample Clock:Rate"](reference=w695, error in=w696) -> (reference out=w694:refnum<k21>, error out=w697:errorcluster)  [unwired: 1 out]
            n297 = property class="DAQmx Timing" props=["Sample Clock:Rate"](reference=w698, error in=w699) -> (reference out=w700:refnum<k21>, error out=w701:errorcluster)  [unwired: 1 out]
            n298 = call "Get Terminal Name with Device Prefix.vi"("error in (no error)"=w701, "Local Terminal Name"="ai/StartTrigger" ("terminal"), "task/channels in"=w700) -> ("error out"=w671:errorcluster, "Terminal Name with Device Prefix"=w693:tag, "task out"=w669:refnum<k21>)  [unwired: 6 in]
            n299 = call-poly <vilib>:"DAQmx Trigger.vi"("task/channels in"=w694, "source"=w693, "error in"=w697) -> ("task out"=w667:refnum<k21>, "error out"=w664:errorcluster)  [unwired: 11 in]
            n300 = call <vilib>:"DAQmx Start Task.vi"("task/channels in"=w669, "error in"=w671) -> ("task out"=w668:refnum<k21>, "error out"=w670:errorcluster)  [unwired: 12 in]
            n301 = call <vilib>:"DAQmx Start Task.vi"("task/channels in"=w667, "error in"=w664) -> ("task out"=w666:refnum<k21>, "error out"=w665:errorcluster)  [unwired: 12 in]
            n302 = Initialize Array(w659, w659) -> ()  [unwired: 1 out]
            n303 = while {
              tunnel: w668 -> [w736]
              tunnel: w670 -> [w735]
              tunnel: w666 -> [w725]
              tunnel: w665 -> [w724]
              tunnel: [w734] -> w677
              tunnel: [w733] -> w676
              shift-right: [w710] -> w660
              shift-left: w663 -> [w715]
              tunnel: [w723] -> w658
              tunnel: [w722] -> w657
              tunnel: w654 -> [w706]
              i -> [w721]
              stop <- w711 stop-if-true
              w719 = 5e-05
              n304 = Absolute Value(x="Setpoint") -> (abs(x)=w702:dbl)
              n305 = call-poly <vilib>:"DAQmx Read.vi"("task/channels in"=w736, "error in"=w735) -> ("task out"=w734:refnum<k21>, "data"=w705:dbl, "error out"=w733:errorcluster)  [unwired: 11 in]
              n306 = Absolute Value(x=w705) -> (abs(x)=w704:dbl)
              n307 = local read "Bias Offset Correct"() -> (w707:dbl)
              n308 = Bundle("Proportional Gain"="Proportional Gain", "Integral Gain"="Integral Gain", "Differential Gain"="Differential Gain") -> (w726:T3)  [unwired: 1 in]
              n309 = local write "Waveform Chart"(w705) -> ()
              n310 = Bundle(10, -10) -> (w730:cluster{i32, i32})  [unwired: 1 in]
              n311 = call-poly "PID.vi"("output range"=w730, "dt (s)"=w719, "PID gains"=w726, "process variable"=w704, "setpoint"=w702) -> ("output"=w718:dbl)  [unwired: 5 in, 1 out]
              n312 = Add(x=w706, y=w707) -> (x+y=w708:dbl)
              n313 = Less?(x=w721, y=1000) -> (x < y?=w716:bool)
              n314 = call-poly "PID Output Rate Limiter.vi"("reinitialize? (F)"=w716, "dt (s)"=w719, "output rate (EGU/min)"="Piezo Delta rate", "initial output"=w715, "input (controller output)"=w718) -> ("output"=w710:dbl)  [unwired: 3 in, 1 out]
              n315 = local write "Piezo Control"(w710) -> ()
              n316 = Build Array(w708, w710) -> (w709:dbl[])
              n317 = local read "Sweep Bias"() -> (w714:bool)
              n318 = local read "PID"() -> (w712:bool)
              n319 = call-poly <vilib>:"DAQmx Write.vi"("task/channels in"=w725, "data"=w709, "error in"=w724) -> ("task out"=w723:refnum<k21>, "error out"=w722:errorcluster)  [unwired: 10 in, 1 out]
              n320 = Not(x=w712) -> (.not. x?=w713:bool)
              n321 = Compound Arithmetic op=OR(w714, w713) -> (w711:bool)
            }
            n322 = call <vilib>:"DAQmx Clear Task.vi"("task in"=w658, "error in"=w657) -> ("error out"=w674:errorcluster)  [unwired: 13 in]
            n323 = call <vilib>:"DAQmx Clear Task.vi"("task in"=w677, "error in"=w676) -> ("error out"=w675:errorcluster)  [unwired: 13 in]
            n324 = Merge Errors(w675, w674) -> (w672:errorcluster)
            n325 = call <vilib>:"General Error Handler.vi"("type of dialog (OK msg:1)"=w673, "error in (no error)"=w672) -> ()  [unwired: 9 in, 5 out]
          }
        }
      }
    }
  }
